vi "Serial_Read_Write.vi"(8 "error in (no error)":errorcluster, 11 "VISA resource name":refnum<visa-resource-name>="ControlBoard") -> (0 "error out":errorcluster, 3 "VISA resource name out":refnum<visa-resource-name>)   [LabVIEW 2022 SP3]
panel:
  in  "Read Byte Control":u32
  out "Serial Settings:Number of Bytes at Serial Port":u32
  out "read buffer":string
  out "return count":u32
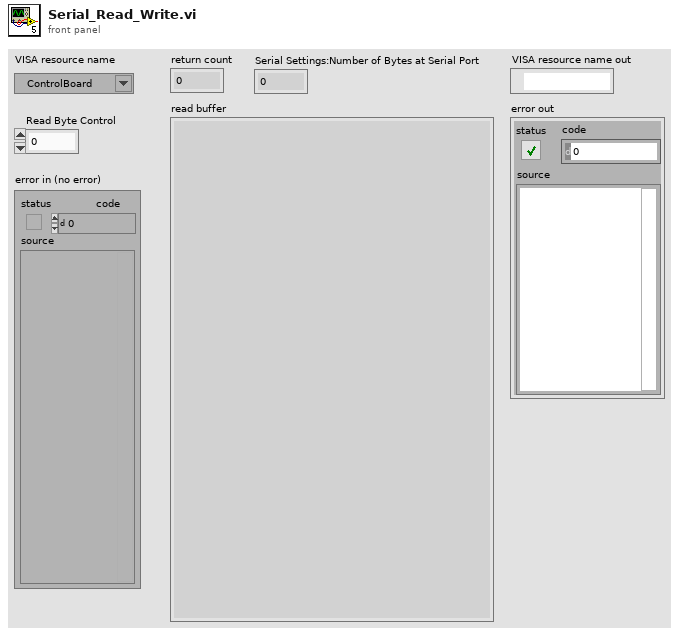
[diagram p1: front panel]
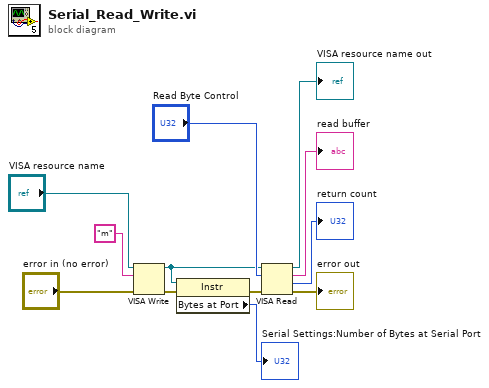
[diagram p0: block diagram]
diagram:
  n1 = VISA Write(VISA resource name="VISA resource name", write buffer="m", error in (no error)="error in (no error)") -> (VISA resource name out=w4:refnum<visa-resource-name>, error out=w2:errorcluster)  [unwired: 1 out]
  n2 = property class="Instr"(reference=w4, error in=w2) -> (error out=w1:errorcluster, "Bytes at Port"=→"Serial Settings:Number of Bytes at Serial Port":u32)  [unwired: 1 out]
  n3 = VISA Read(VISA resource name=w4, byte count="Read Byte Control", error in (no error)=w1) -> (VISA resource name out=→"VISA resource name out":refnum<visa-resource-name>, read buffer=→"read buffer":string, return count=→"return count":u32, error out=→"error out":errorcluster)
